vi "Check_Trigger_and_stop.vi"(7 "DAQ_VI":refnum<vi>, 8 "error in (no error)":errorcluster, 10 "Command_Message_in":T1, 11 "Command_queue_in":T2) -> (0 "error out":errorcluster, 2 "Command_Message_out":T1)   [LabVIEW 2024]
uses:
  Command_Message.ctl
  Command_Queue.ctl
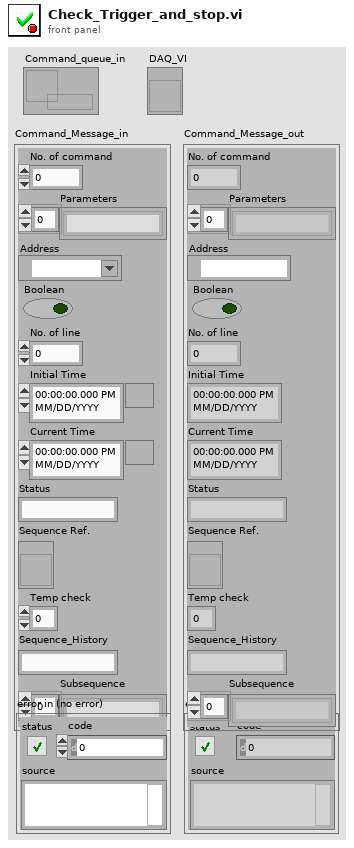
[diagram p1: front panel]
types:
  T1 = typedef "Command_Message.ctl" = cluster{"No. of command":i32, "Parameters":string[], "Address":refnum<visa-resource-name>, "Boolean":bool, "No. of line":i32, "Initial Time":timestamp, "Current Time":timestamp, "Status":string, "Sequence Ref.":refnum<vi>, "Temp check":i32, "Sequence_History":string, "Subsequence":string[]}
  T2 = typedef "Command_Queue.ctl" = refnum<queue>
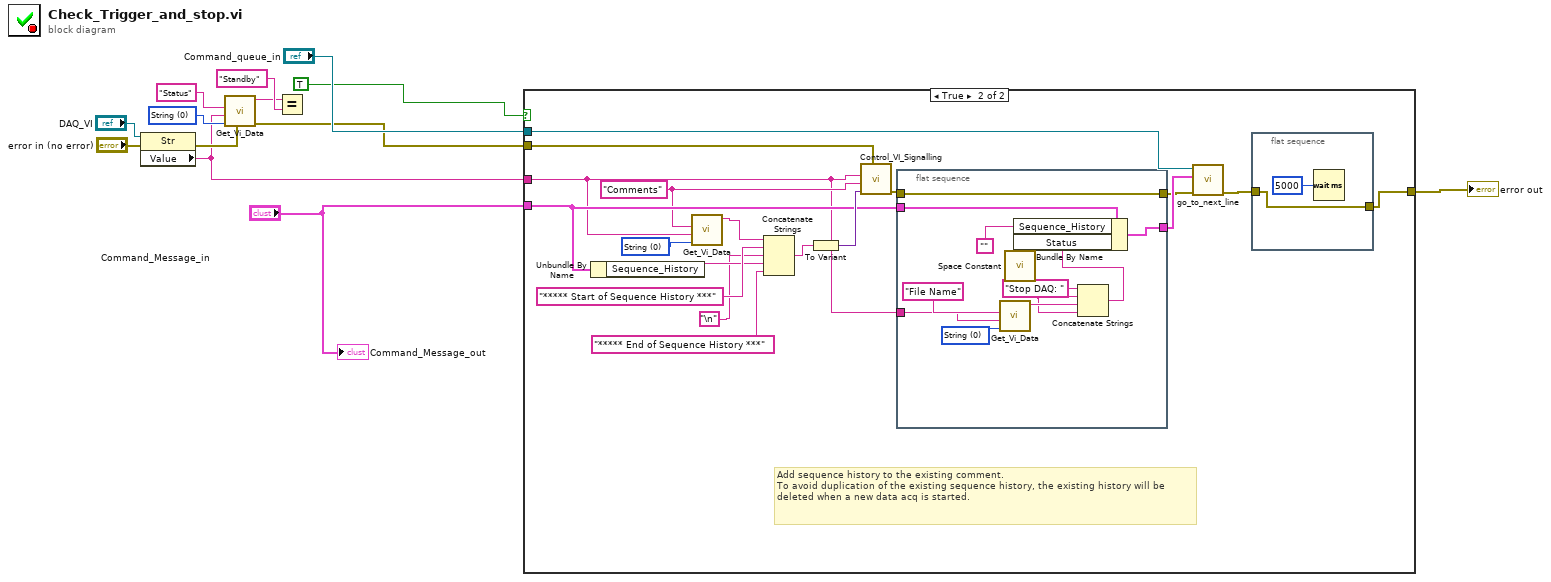
[diagram p0: block diagram]
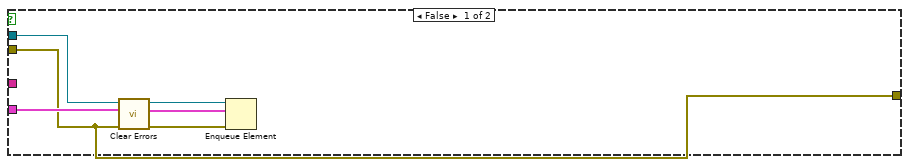
[diagram p2: hidden frame]
diagram:
  w8 = u16 0 items=["String", "Double", "Boolean", "Variant"] ("Data Type")
  n1 = property on="Property Node" class="Str"(reference="DAQ_VI", error in="error in (no error)") -> (error out=w6:errorcluster, "Value"=w5:string)  [unwired: 1 out]
  n2 = call "Get_Vi_Data.vi"("error in (no error) 2"=w6, "Data Type"=w8, "VI name"=w5, "Control Name"="Status") -> ("error out"=w4:errorcluster, "Data (String)"=w2:string)  [unwired: 3 in, 3 out]
  n3 = Equal?(x=w2, y="Standby") -> ()  [unwired: 1 out]
  n4 = case shown="True" TRUE {
    tunnel: "Command_queue_in" -> [w16 w31]
    tunnel: "Command_Message_in" -> [w17 w30]
    tunnel: w4 -> [w14 w32]
    tunnel: [w14 w25] -> w11
    tunnel: w5 -> [_ w18]
    frame False {
      n5 = call <vilib>:"Clear Errors.vi"("error in (no error)"=w14) -> ("error out"=w15:errorcluster)  [unwired: 5 in, 1 out]
      n6 = Enqueue Element(queue=w16, element=w17, error in (no error)=w15) -> ()  [unwired: 1 in, 3 out]
    }
    frame True {
      w23 = u16 0 items=["String", "Double", "Boolean", "Variant"] ("Data Type")
      w24 = "Comments" ("Control Name")
      # "Add sequence history to the existing comment.\nTo avoid duplication of the existing sequence history, the existing history will be\ndeleted when a new data acq is started."
      n7 = Unbundle By Name(w30) -> ("Sequence_History"=w20:string)
      n8 = call "Get_Vi_Data.vi"("Data Type"=w23, "VI name"=w18, "Control Name"=w24) -> ("Data (String)"=w22:string)  [unwired: 4 in, 4 out]
      n9 = Concatenate Strings(w22, "***** Start of Sequence History ***" ("string"), "\n", w20, "***** End of Sequence History ***" ("string")) -> (w34:string)
      n10 = To Variant(anything=w34) -> (Variant=w35:variant)
      n11 = call "Control_VI_Signalling.vi"("error in (no error)"=w32, "Input Value"=w35, "Control Name"=w24, "Target VI name"=w18) -> ("error out"=w28:errorcluster)  [unwired: 7 in]
      n12 = flat-sequence {
        tunnel: w30 -> [w48]
        tunnel: [w47] -> w29
        tunnel: w28 -> [w46]
        tunnel: [w46] -> w27
        tunnel: w18 -> [w43]
        frame #0 {
          w44 = u16 0 items=["String", "Double", "Boolean", "Variant"] ("Data Type")
          n13 = call "Get_Vi_Data.vi"("Data Type"=w44, "VI name"=w43, "Control Name"="File Name") -> ("Data (String)"=w42:string)  [unwired: 4 in, 4 out]
          n14 = call <vilib>:"Space Constant.vi"() -> ("String"=w41:string)
          n15 = Concatenate Strings("Stop DAQ: " ("string"), w41, w42, w41) -> (w39:string)
          n16 = Bundle By Name(cluster=w48, "Sequence_History"="", "Status"=w39) -> (w47:T1)
        }
      }
      n17 = call "go_to_next_line.vi"("error in (no error)"=w27, "Message_command in"=w29, "Command Queue in"=w31) -> ("error out"=w26:errorcluster)  [unwired: 7 in, 1 out]
      n18 = flat-sequence {
        tunnel: w26 -> [w36]
        tunnel: [w36] -> w25
        frame #0 {
          n19 = Wait (ms)(milliseconds to wait=u32 5000) -> ()  [unwired: 1 out]
        }
      }
    }
  }
  "error out" <- w11
  "Command_Message_out" <- "Command_Message_in"
